vi "Stale Values.vi"(8 "error in (no error)":errorcluster, 11 "MB Master in":refnum<class "MB Slave Simulator Base.lvclass">) -> (0 "error out":errorcluster)   [LabVIEW 2021, in "MB Slave Simulator Base.lvclass"]
uses:
  MB Slave Simulator Base.lvclass
  MB Slave Simulator Base.lvclass/MB Slave Simulator Base.ctl
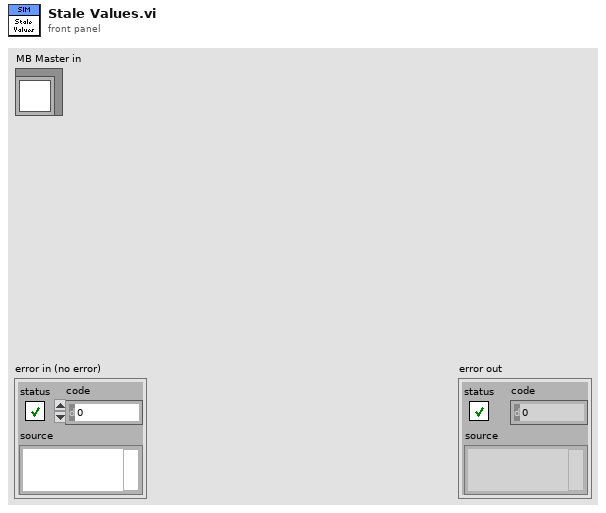
[diagram p1: front panel]
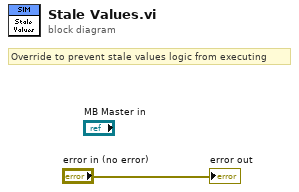
[diagram p0: block diagram]
diagram:
  # "Override to prevent stale values logic from executing"
  "error out" <- "error in (no error)"
